vi "dxf提取圆坐标点.vi"(11 "字符串":string) -> (3 "输出数组":cluster{"x":dbl, "y":dbl, "r":dbl}[](array[cluster]))   [LabVIEW 2014]
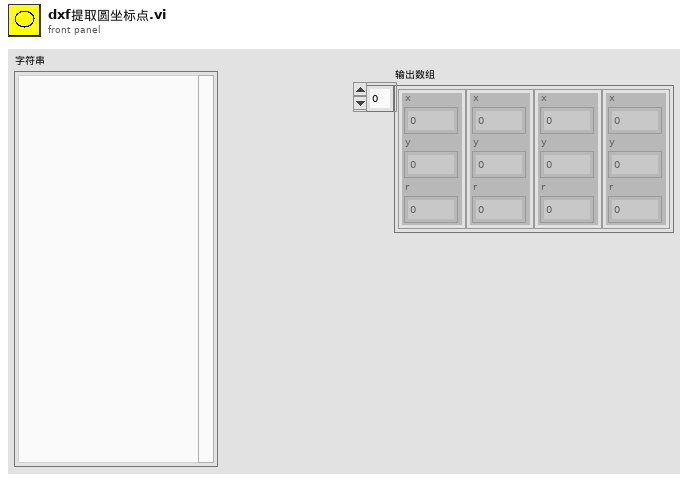
[diagram p1: front panel]
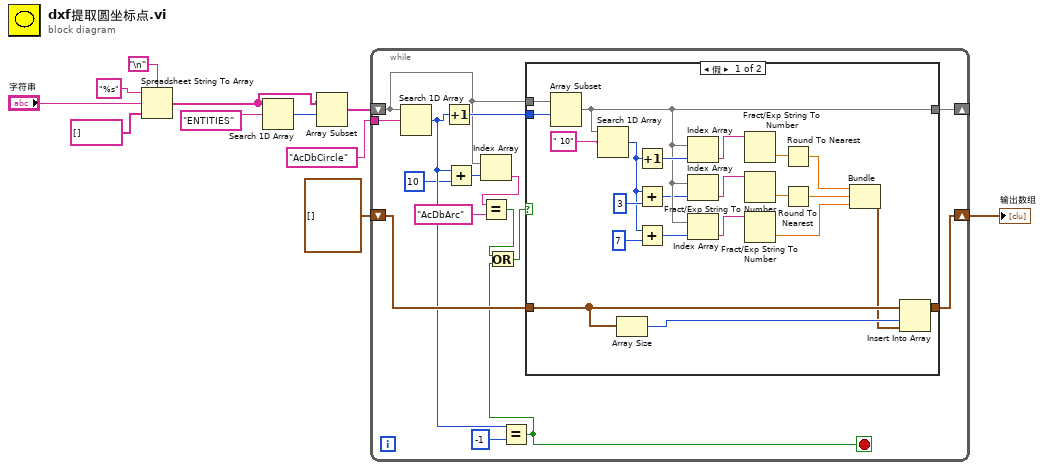
[diagram p0: block diagram]
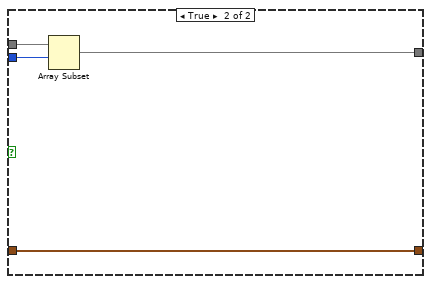
[diagram p2: hidden frame]
diagram:
  n1 = Spreadsheet String To Array(delimiter (Tab)="\n", format string="%s" ("格式字符串"), spreadsheet string="字符串", array type (2D Dbl)=string[] [] ("数组类型(2D Dbl)")) -> (array=w5:string[])
  n2 = Search 1D Array(1D array=w5, element="ENTITIES" ("元素")) -> (index of element=w6:i32)  [unwired: 1 in]
  n3 = Array Subset(array=w5, index=w6) -> (w4:string[])  [unwired: 1 in]
  n4 = while {
    tunnel: "AcDbCircle" ("元素") -> [w26]
    shift-right: [w23] -> _
    shift-left: w4 -> [w20]
    shift-right: [w22] -> w2
    shift-left: cluster{dbl, dbl, dbl}[] [] -> [w21]
    stop <- w12 stop-if-true
    n5 = Search 1D Array(1D array=w20, element=w26) -> (index of element=w18:i32)  [unwired: 1 in]
    n6 = Increment(x=w18) -> (x+1=w24:i32)
    n7 = Add(x=w18, y=10) -> (x+y=w19:i32)
    n8 = Index Array(array=w20, index=w19) -> (element=w16:string)
    n9 = Equal?(x=w16, y="AcDbArc" ("元素")) -> (x = y?=w13:bool)
    n10 = Equal?(x=w18, y=-1) -> (x = y?=w12:bool)
    n11 = Or(x=w13, y=w12) -> (x .or. y?=w14:bool)
    n12 = case shown="假" w14 {
      tunnel: w24 -> [w48 w49]
      tunnel: [w46 w50] -> w23
      tunnel: [w33 w52] -> w22
      tunnel: w21 -> [w32 w52]
      tunnel: w20 -> [w28 w51]
      frame False {
        n13 = Array Subset(array=w28, index=w48) -> (w46:string[])  [unwired: 1 in]
        n14 = Search 1D Array(1D array=w46, element=" 10") -> (index of element=w41:i32)  [unwired: 1 in]
        n15 = Array Size(array=w32) -> (size(s)=w30:i32)
        n16 = Increment(x=w41) -> (x+1=w47:i32)
        n17 = Add(x=w41, y=i8 3) -> (x+y=w45:i32)
        n18 = Add(x=w41, y=i8 7) -> (x+y=w44:i32)
        n19 = Index Array(array=w46, index=w47) -> (element=w40:string)
        n20 = Index Array(array=w46, index=w45) -> (element=w39:string)
        n21 = Index Array(array=w46, index=w44) -> (element=w38:string)
        n22 = Fract/Exp String To Number(string=w40) -> (number=w37:dbl)  [unwired: 3 in, 1 out]
        n23 = Fract/Exp String To Number(string=w39) -> (number=w36:dbl)  [unwired: 3 in, 1 out]
        n24 = Fract/Exp String To Number(string=w38) -> (number=w27:dbl)  [unwired: 3 in, 1 out]
        n25 = Round To Nearest(number=w37) -> (nearest integer value=w35:dbl)
        n26 = Round To Nearest(number=w36) -> (nearest integer value=w34:dbl)
        n27 = Bundle(w35, w34, w27) -> (w29:cluster{dbl, dbl, dbl})  [unwired: 1 in]
        n28 = Insert Into Array(array=w32, index=w30, new element=w29) -> (w33:cluster{dbl, dbl, dbl}[])
      }
      frame True {
        n29 = Array Subset(array=w51, index=w49) -> (w50:string[])  [unwired: 1 in]
      }
    }
  }
  "输出数组" <- w2
